vi "Allocate Buffers.vi"(10 "Timestamps and Lengths Size (128)":i32=128, 11 "capture_size (524288)":i32=524288) -> (2 "Timestamps and Lengths Buffer":T1, 3 "capture_data buffer":string)   [LabVIEW 2025, in "Automotive Ethernet Bus Monitor UI.lvlib" / "lvwpcap.lvlib"]
uses:
  lvwpcap.lvlib
  types/Capture Legnths.ctl
  types/Timestamps and Lengths.ctl
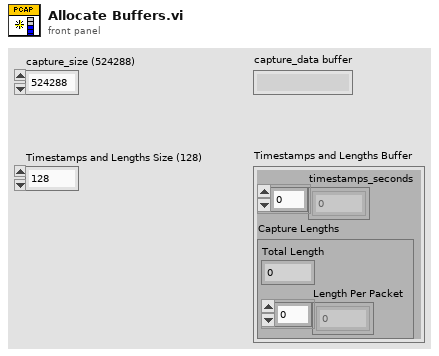
[diagram p1: front panel]
types:
  T1 = typedef "Automotive Ethernet Bus Monitor UI.lvlib/lvwpcap.lvlib/Timestamps and Lengths.ctl" = cluster{"timestamps_seconds":dbl[], "Capture Lengths":T2}
  T2 = typedef "Automotive Ethernet Bus Monitor UI.lvlib/lvwpcap.lvlib/Capture Legnths.ctl" = cluster{"Total Length":u32, "Length Per Packet":u32[]}
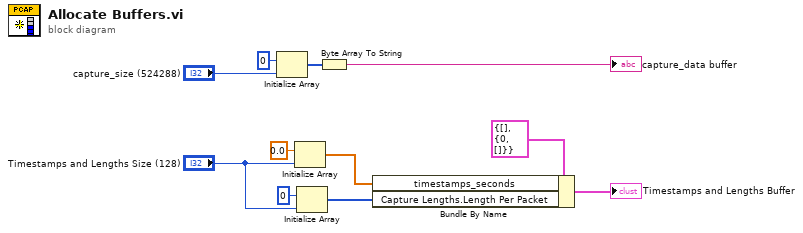
[diagram p0: block diagram]
diagram:
  n1 = Initialize Array(u8 0, "capture_size (524288)") -> (w9:u8[])
  n2 = Initialize Array(0.0, "Timestamps and Lengths Size (128)") -> (w4:dbl[])
  n3 = Initialize Array(u32 0, "Timestamps and Lengths Size (128)") -> (w1:u32[])
  n4 = Byte Array To String(unsigned byte array=w9) -> (string=→"capture_data buffer":string)
  n5 = Bundle By Name(cluster=T1 {"timestamps_seconds"=[], "Capture Lengths"={"Total Length"=0, "Length Per Packet"=[]}} ("Timestamps and Lengths Buffer"), "timestamps_seconds"=w4, "Capture Lengths.Length Per Packet"=w1) -> (→"Timestamps and Lengths Buffer":T1)
